vi "Argus Cal Helper.vi"() -> ()   [LabVIEW 2020]
doc: "Demonstrates how to use the DC Voltage Output Function to force an output voltage. This example initializes a session, configures the Output Function, Sense, Autorange, Voltage Level and Current Limit, initiates generation, waits for a specified delay, and measures the voltage and current output. This example uses Single Point source mode."
uses:
  <instrlib>/niDCPower/nidcpower.llb/niDCPower Sense.ctl
  <instrlib>/niDCPower/nidcpower.llb/niDCPower Output Function.ctl
  <instrlib>/niDCPower/nidcpower.llb/niDCPower Source Mode.ctl
  <instrlib>/niDCPower/nidcpower.llb/niDCPower Wait For Event - Event.ctl
  <instrlib>/niDCPower/nidcpower.llb/niDCPower Configure Digital Edge Source Trigger With Channels.vi
  <instrlib>/niDCPower/nidcpower.llb/niDCPower Configure Digital Edge Measure Trigger With Channels.vi
panel:
  in  "Voltage Sense":T1=1009 items=["Local"=1008, "Remote"=1009]
  in  "Voltage Sense 2":T1=1008 caption="Voltage Sense" items=["Local"=1008, "Remote"=1009]
  in  "Aperture Time (Sec) 2":dbl=1.0 caption="Aperture Time (Sec)" format="%.3p"
  in  "Aperture Time (Sec)":dbl=1.0 format="%.3p"
  out "In compliance 2":bool[](array[boolean]) caption="In Compliance"
  out "In compliance":bool[](array[boolean]) caption="In Compliance"
  in  "Source Delay (Sec)":dbl=1.0 format="%.3p"
  out "Voltage Measurement":dbl
  out "Current Measurement":dbl
  in  "Current Limit Range":dbl=1.5 format="%.3p"
  in  "Voltage Level Range":dbl=12.0 format="%.5p"
  in  "Current Limit":dbl=1.5 format="%.3p"
  in  "Voltage Level":dbl=12.0 format="%.5p"
  in  "Channel Name":string="0"
  in  "Resource Name":refnum<k15>="Dev1"
  in  "Source Delay (Sec) 2":dbl=1.0 caption="Source Delay (Sec)" format="%.3p"
  out "Voltage Measurement 2":dbl caption="Voltage Measurement"
  out "Current Measurement 2":dbl caption="Current Measurement"
  in  "Voltage Limit Range":dbl=20.0 format="%.5p"
  in  "Current Level Range":dbl=1.0 format="%.3p"
  in  "Voltage Limit":dbl=20.0 format="%.5p"
  in  "Current Level":dbl=1.0 format="%.3p"
  in  "Channel Name 2":string="0" caption="Channel Name"
  in  "Resource Name 2":refnum<k15>="Dev1" caption="Resource Name"
  # "Overview: \nRequirements: NI-DCPower\nInstructions:\n1. Select the appropriate device in the Resource Name control.\n2. Configure the parameters of the DC Voltage signal you'd like to output.\n3. Run the VI."
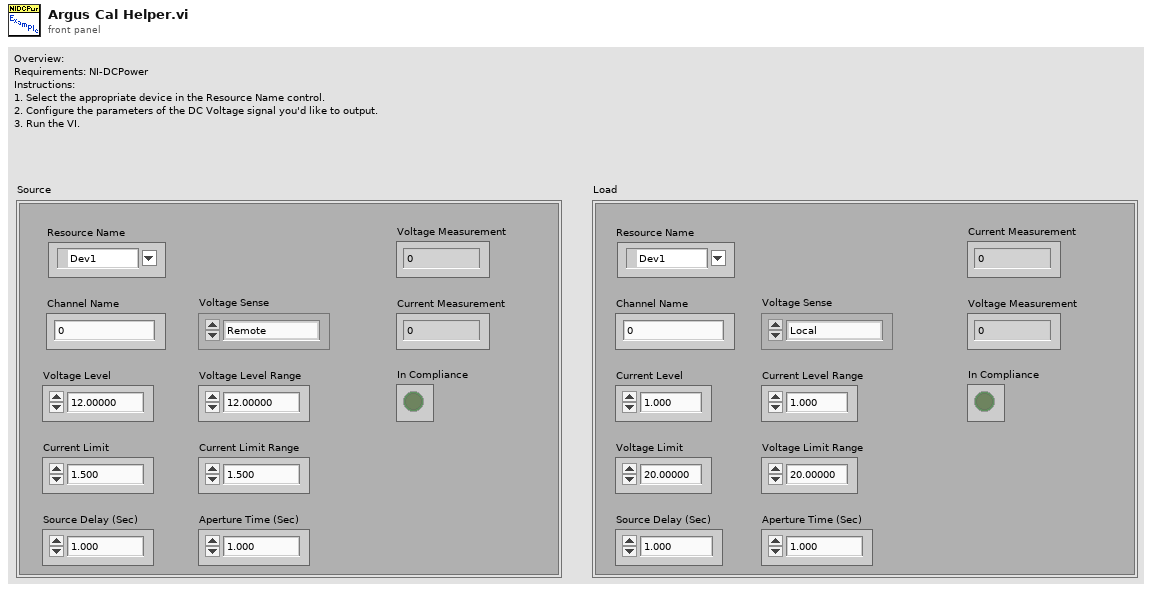
[diagram p1: front panel]
types:
  T1 = typedef "niDCPower Sense.ctl" = i32
  T2 = typedef "niDCPower Wait For Event - Event.ctl" = i32
  T3 = typedef "niDCPower Output Function.ctl" = i32
  T4 = typedef "niDCPower Source Mode.ctl" = i32
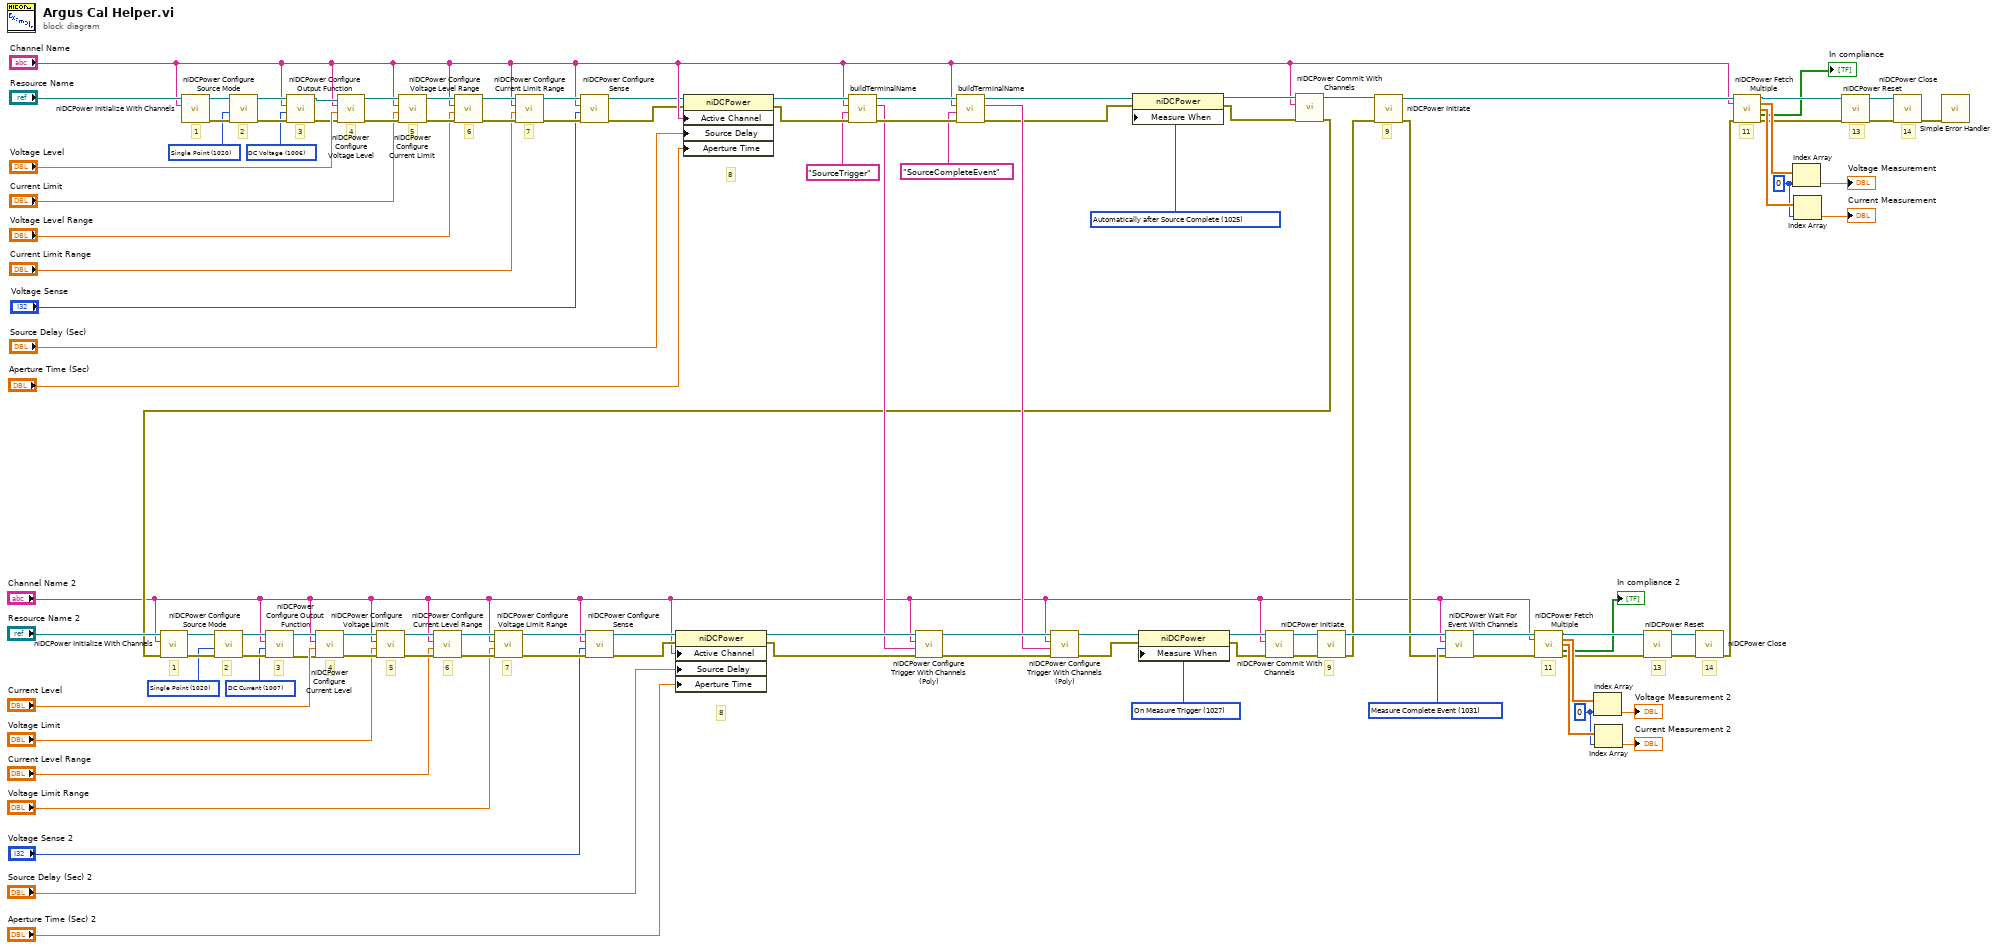
[diagram p0: block diagram]
diagram:
  w35 = T2 1031 items=["Source Complete Event"=1030, "Measure Complete Event"=1031, "Sequence Iteration Complete Event"=1032, "Sequence Engine Done Event"=1033, "Pulse Complete Event"=1051, "Ready For Pulse Trigger Event"=1052] ("event")
  w37 = 1027 items=["Automatically after Source Complete"=1025, "On Demand"=1026, "On Measure Trigger"=1027] ("Measurement:Advanced:Measure When")
  w40 = 1025 items=["Automatically after Source Complete"=1025, "On Demand"=1026, "On Measure Trigger"=1027] ("Measurement:Advanced:Measure When")
  w55 = T3 1007 items=["DC Voltage"=1006, "DC Current"=1007, "Pulse Voltage"=1049, "Pulse Current"=1050] ("output function")
  w61 = 0 ("index")
  w70 = T4 1020 items=["Single Point"=1020, "Sequence"=1021] ("source mode")
  w82 = T3 1006 items=["DC Voltage"=1006, "DC Current"=1007, "Pulse Voltage"=1049, "Pulse Current"=1050] ("output function")
  w88 = 0 ("index")
  w97 = T4 1020 items=["Single Point"=1020, "Sequence"=1021] ("source mode")
  # "14"
  # "8"
  # "11"
  # "7"
  # "6"
  # "2"
  # "3"
  # "13"
  # "9"
  # "5"
  # "4"
  # "1"
  # "14"
  # "9"
  # "11"
  # "7"
  # "6"
  # "2"
  # "3"
  # "13"
  # "8"
  # "5"
  # "4"
  # "1"
  n1 = call <instrlib>:"niDCPower Initialize With Channels.vi"("channels"="Channel Name", "resource name"="Resource Name") -> ("error out"=w101:errorcluster, "instrument handle out"=w100:refnum<k15>)  [unwired: 3 in, 5 out]
  n2 = call <instrlib>:"niDCPower Configure Source Mode.vi"("error in (no error)"=w101, "source mode"=w97, "instrument handle"=w100) -> ("error out"=w99:errorcluster, "instrument handle out"=w98:refnum<k15>)  [unwired: 7 out]
  n3 = call <instrlib>:"niDCPower Configure Output Function.vi"("error in (no error)"=w99, "output function"=w82, "channel name"="Channel Name", "instrument handle"=w98) -> ("error out"=w83:errorcluster, "instrument handle out"=w84:refnum<k15>)  [unwired: 6 out]
  n4 = call <instrlib>:"niDCPower Configure Voltage Level.vi"("error in (no error)"=w83, "voltage level"="Voltage Level", "channel name"="Channel Name", "instrument handle"=w84) -> ("error out"=w107:errorcluster, "instrument handle out"=w108:refnum<k15>)  [unwired: 6 out]
  n5 = call <instrlib>:"niDCPower Configure Current Limit.vi"("error in (no error)"=w107, "current limit"="Current Limit", "channel name"="Channel Name", "instrument handle"=w108) -> ("error out"=w96:errorcluster, "instrument handle out"=w95:refnum<k15>)  [unwired: 1 in, 5 out]
  n6 = call <instrlib>:"niDCPower Configure Voltage Level Range.vi"("error in (no error)"=w96, "voltage level range"="Voltage Level Range", "channel name"="Channel Name", "instrument handle"=w95) -> ("error out"=w94:errorcluster, "instrument handle out"=w93:refnum<k15>)  [unwired: 6 out]
  n7 = call <instrlib>:"niDCPower Configure Current Limit Range.vi"("error in (no error)"=w94, "current limit range"="Current Limit Range", "channel name"="Channel Name", "instrument handle"=w93) -> ("error out"=w12:errorcluster, "instrument handle out"=w11:refnum<k15>)  [unwired: 6 out]
  n8 = call <instrlib>:"niDCPower Configure Sense.vi"("error in (no error)"=w12, "sense"="Voltage Sense", "channel name"="Channel Name", "instrument handle"=w11) -> ("error out"=w7:errorcluster, "instrument handle out"=w8:refnum<k15>)  [unwired: 6 in]
  n9 = property class="niDCPower"(reference=w8, error in=w7, "Active Channel"="Channel Name", "Source Delay"="Source Delay (Sec)", "Aperture Time"="Aperture Time (Sec)") -> (reference out=w54:refnum<k15>, error out=w53:errorcluster)
  n10 = call "buildTerminalName.vi"("error in (no error)"=w53, "Local Terminal Name"="SourceTrigger", "Channel Name"="Channel Name", "session handle"=w54) -> ("error IO"=w51:errorcluster, "Fully Qualified Terminal Name"=w46:string, "session handle 2"=w50:refnum<k15>)  [unwired: 5 in]
  n11 = call "buildTerminalName.vi"("error in (no error)"=w51, "Local Terminal Name"="SourceCompleteEvent", "Channel Name"="Channel Name", "session handle"=w50) -> ("error IO"=w41:errorcluster, "Fully Qualified Terminal Name"=w43:string, "session handle 2"=w42:refnum<k15>)  [unwired: 5 in]
  n12 = property class="niDCPower"(reference=w42, error in=w41, "Measure When"=w40) -> (reference out=w34:refnum<k15>, error out=w33:errorcluster)
  n13 = call <instrlib>:"niDCPower Commit With Channels.vi"("error in (no error)"=w33, "channel name"="Channel Name", "instrument handle"=w34) -> ("error out"=w30:errorcluster, "instrument handle out"=w32:refnum<k15>)  [unwired: 7 in]
  n14 = call <instrlib>:"niDCPower Initialize With Channels.vi"("error in (no error)"=w30, "channels"="Channel Name 2", "resource name"="Resource Name 2") -> ("error out"=w74:errorcluster, "instrument handle out"=w73:refnum<k15>)  [unwired: 2 in, 5 out]
  n15 = call <instrlib>:"niDCPower Configure Source Mode.vi"("error in (no error)"=w74, "source mode"=w70, "instrument handle"=w73) -> ("error out"=w72:errorcluster, "instrument handle out"=w71:refnum<k15>)  [unwired: 7 out]
  n16 = call <instrlib>:"niDCPower Configure Output Function.vi"("error in (no error)"=w72, "output function"=w55, "channel name"="Channel Name 2", "instrument handle"=w71) -> ("error out"=w57:errorcluster, "instrument handle out"=w56:refnum<k15>)  [unwired: 6 out]
  n17 = call <instrlib>:"niDCPower Configure Current Level.vi"("error in (no error)"=w57, "current level"="Current Level", "channel name"="Channel Name 2", "instrument handle"=w56) -> ("error out"=w79:errorcluster, "instrument handle out"=w80:refnum<k15>)  [unwired: 6 out]
  n18 = call <instrlib>:"niDCPower Configure Voltage Limit.vi"("error in (no error)"=w79, "voltage limit"="Voltage Limit", "channel name"="Channel Name 2", "instrument handle"=w80) -> ("error out"=w69:errorcluster, "instrument handle out"=w68:refnum<k15>)  [unwired: 6 out]
  n19 = call <instrlib>:"niDCPower Configure Current Level Range.vi"("error in (no error)"=w69, "current level range"="Current Level Range", "channel name"="Channel Name 2", "instrument handle"=w68) -> ("error out"=w67:errorcluster, "instrument handle out"=w66:refnum<k15>)  [unwired: 6 out]
  n20 = call <instrlib>:"niDCPower Configure Voltage Limit Range.vi"("error in (no error)"=w67, "voltage limit range"="Voltage Limit Range", "channel name"="Channel Name 2", "instrument handle"=w66) -> ("error out"=w4:errorcluster, "instrument handle out"=w3:refnum<k15>)  [unwired: 6 out]
  n21 = call <instrlib>:"niDCPower Configure Sense.vi"("error in (no error)"=w4, "sense"="Voltage Sense 2", "channel name"="Channel Name 2", "instrument handle"=w3) -> ("error out"=w6:errorcluster, "instrument handle out"=w5:refnum<k15>)  [unwired: 6 in]
  n22 = property class="niDCPower"(reference=w5, error in=w6, "Active Channel"="Channel Name 2", "Source Delay"="Source Delay (Sec) 2", "Aperture Time"="Aperture Time (Sec) 2") -> (reference out=w48:refnum<k15>, error out=w47:errorcluster)
  n23 = call-poly <instrlib>:"niDCPower Configure Trigger With Channels (Poly).vi"("error in (no error)"=w47, "input terminal"=w46, "channel name"="Channel Name 2", "instrument handle"=w48) -> ("error out"=w45:errorcluster, "instrument handle out"=w44:refnum<k15>)  [unwired: 6 in]
  n24 = call-poly <instrlib>:"niDCPower Configure Trigger With Channels (Poly).vi"("error in (no error)"=w45, "input terminal"=w43, "channel name"="Channel Name 2", "instrument handle"=w44) -> ("error out"=w38:errorcluster, "instrument handle out"=w39:refnum<k15>)  [unwired: 6 in]
  n25 = property class="niDCPower"(reference=w39, error in=w38, "Measure When"=w37) -> (reference out=w24:refnum<k15>, error out=w23:errorcluster)
  n26 = call <instrlib>:"niDCPower Commit With Channels.vi"("error in (no error)"=w23, "channel name"="Channel Name 2", "instrument handle"=w24) -> ("error out"=w21:errorcluster, "instrument handle out"=w22:refnum<k15>)  [unwired: 7 in]
  n27 = call <instrlib>:"niDCPower Initiate.vi"("error in (no error)"=w21, "instrument handle"=w22) -> ("error out"=w29:errorcluster, "instrument handle out"=w36:refnum<k15>)  [unwired: 2 in, 6 out]
  n28 = call <instrlib>:"niDCPower Initiate.vi"("error in (no error)"=w29, "instrument handle"=w32) -> ("error out"=w28:errorcluster, "instrument handle out"=w31:refnum<k15>)  [unwired: 2 in, 6 out]
  n29 = call <instrlib>:"niDCPower Wait For Event With Channels.vi"("error in (no error)"=w28, "event"=w35, "channel name"="Channel Name 2", "instrument handle"=w36) -> ("error out"=w26:errorcluster, "instrument handle out"=w27:refnum<k15>)  [unwired: 6 in]
  n30 = call <instrlib>:"niDCPower Fetch Multiple.vi"("instrument handle"=w27, "channel name"="Channel Name 2", "error in (no error)"=w26) -> ("instrument handle out"=w17:refnum<k15>, "voltage measurements"=w63:dbl[], "current measurements"=w62:dbl[], "in compliance"=→"In compliance 2":bool[], "error out"=w16:errorcluster)  [unwired: 7 in, 1 out]
  n31 = Index Array(array=w63, index=w61) -> (element=→"Voltage Measurement 2":dbl)
  n32 = Index Array(array=w62, index=w61) -> (element=→"Current Measurement 2":dbl)
  n33 = call <instrlib>:"niDCPower Reset.vi"("error in (no error)"=w16, "instrument handle"=w17) -> ("error out"=w76:errorcluster, "instrument handle out"=w77:refnum<k15>)  [unwired: 2 in, 6 out]
  n34 = call <instrlib>:"niDCPower Close.vi"("error in (no error)"=w76, "instrument handle"=w77) -> ("error out"=w25:errorcluster)  [unwired: 9 out]
  n35 = call <instrlib>:"niDCPower Fetch Multiple.vi"("instrument handle"=w31, "channel name"="Channel Name", "error in (no error)"=w25) -> ("instrument handle out"=w20:refnum<k15>, "voltage measurements"=w90:dbl[], "current measurements"=w89:dbl[], "in compliance"=→"In compliance":bool[], "error out"=w19:errorcluster)  [unwired: 7 in, 1 out]
  n36 = Index Array(array=w90, index=w88) -> (element=→"Voltage Measurement":dbl)
  n37 = Index Array(array=w89, index=w88) -> (element=→"Current Measurement":dbl)
  n38 = call <instrlib>:"niDCPower Reset.vi"("error in (no error)"=w19, "instrument handle"=w20) -> ("error out"=w104:errorcluster, "instrument handle out"=w105:refnum<k15>)  [unwired: 2 in, 6 out]
  n39 = call <instrlib>:"niDCPower Close.vi"("error in (no error)"=w104, "instrument handle"=w105) -> ("error out"=w103:errorcluster)  [unwired: 9 out]
  n40 = call <vilib>:"Simple Error Handler.vi"("error in (no error)"=w103) -> ()  [unwired: 1 in, 8 out]
